vi "Write Hardware Queue.vi"(8 "error in (no error)":errorcluster, 10 "Actor Framework:Message Enqueuer":refnum<class "Message Enqueuer.lvclass">, 11 "Meter Measurement in":refnum<class "Meter Measurement.lvclass">) -> (0 "error out":errorcluster, 3 "Meter Measurement out":refnum<class "Meter Measurement.lvclass">)   [LabVIEW 2015, in "Meter Measurement.lvclass"]
uses:
  Meter Measurement.lvclass
  <vilib>/ActorFramework/Message Enqueuer/Message Enqueuer.lvclass
  Meter Measurement.lvclass/Meter Measurement.ctl
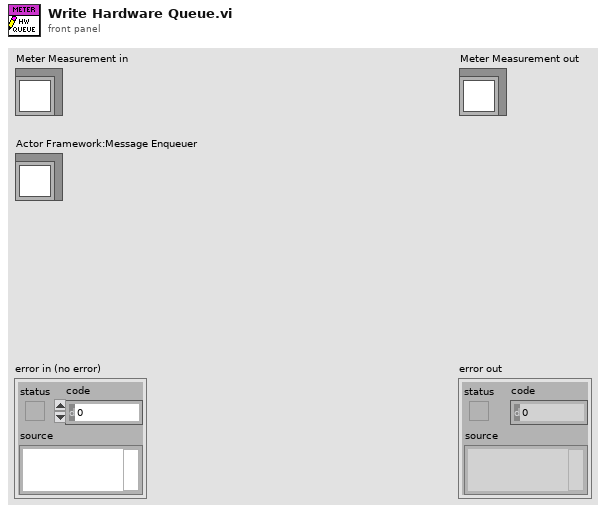
[diagram p1: front panel]
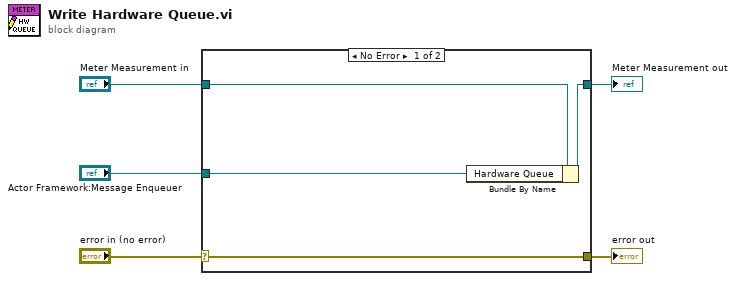
[diagram p0: block diagram]
diagram:
  n1 = case shown="No Error" "error in (no error)" {
    selector: "error in (no error)" -> [w9 w10]
    tunnel: [w9 w10] -> w4
    tunnel: [w7 w11] -> w2
    tunnel: "Meter Measurement in" -> [w8 w11]
    tunnel: "Actor Framework:Message Enqueuer" -> [w6 _]
    frame No Error {
      n2 = Bundle By Name(cluster=w8, "Hardware Queue"=w6) -> (w7:refnum<class "Meter Measurement.lvclass">)
    }
    frame Error {
    }
  }
  "error out" <- w4
  "Meter Measurement out" <- w2
